vi "Trainging_Program_redesign_Alarm.vi"() -> ()   [LabVIEW 2014]
uses:
  <vilib>/Utility/file.llb/Write To Spreadsheet File (I64).vi
  <vilib>/Utility/file.llb/Write To Spreadsheet File (DBL).vi
  NeuroSky_Dll_Call/Debug/NeuroSky_Dll_Call.dll
panel:
  out "큐사인":bool
  out "실험종료":bool=TRUE
  out "icon_온도":bool
  out "icon_자판":bool
  out "icon_침대":bool
  out "icon_기계":bool
  out "icon_응급":bool=TRUE
  out "icon_용변":bool
  out "error out":errorcluster={"status"=TRUE, "code"=10, "source"="Create Folder in Trainging_Set_For_ LDA_Matrix_RSVP.vi<APPEND>\nC:\\Emotion_Research\\_Training_Test(LDA)\\2014-08-30"}
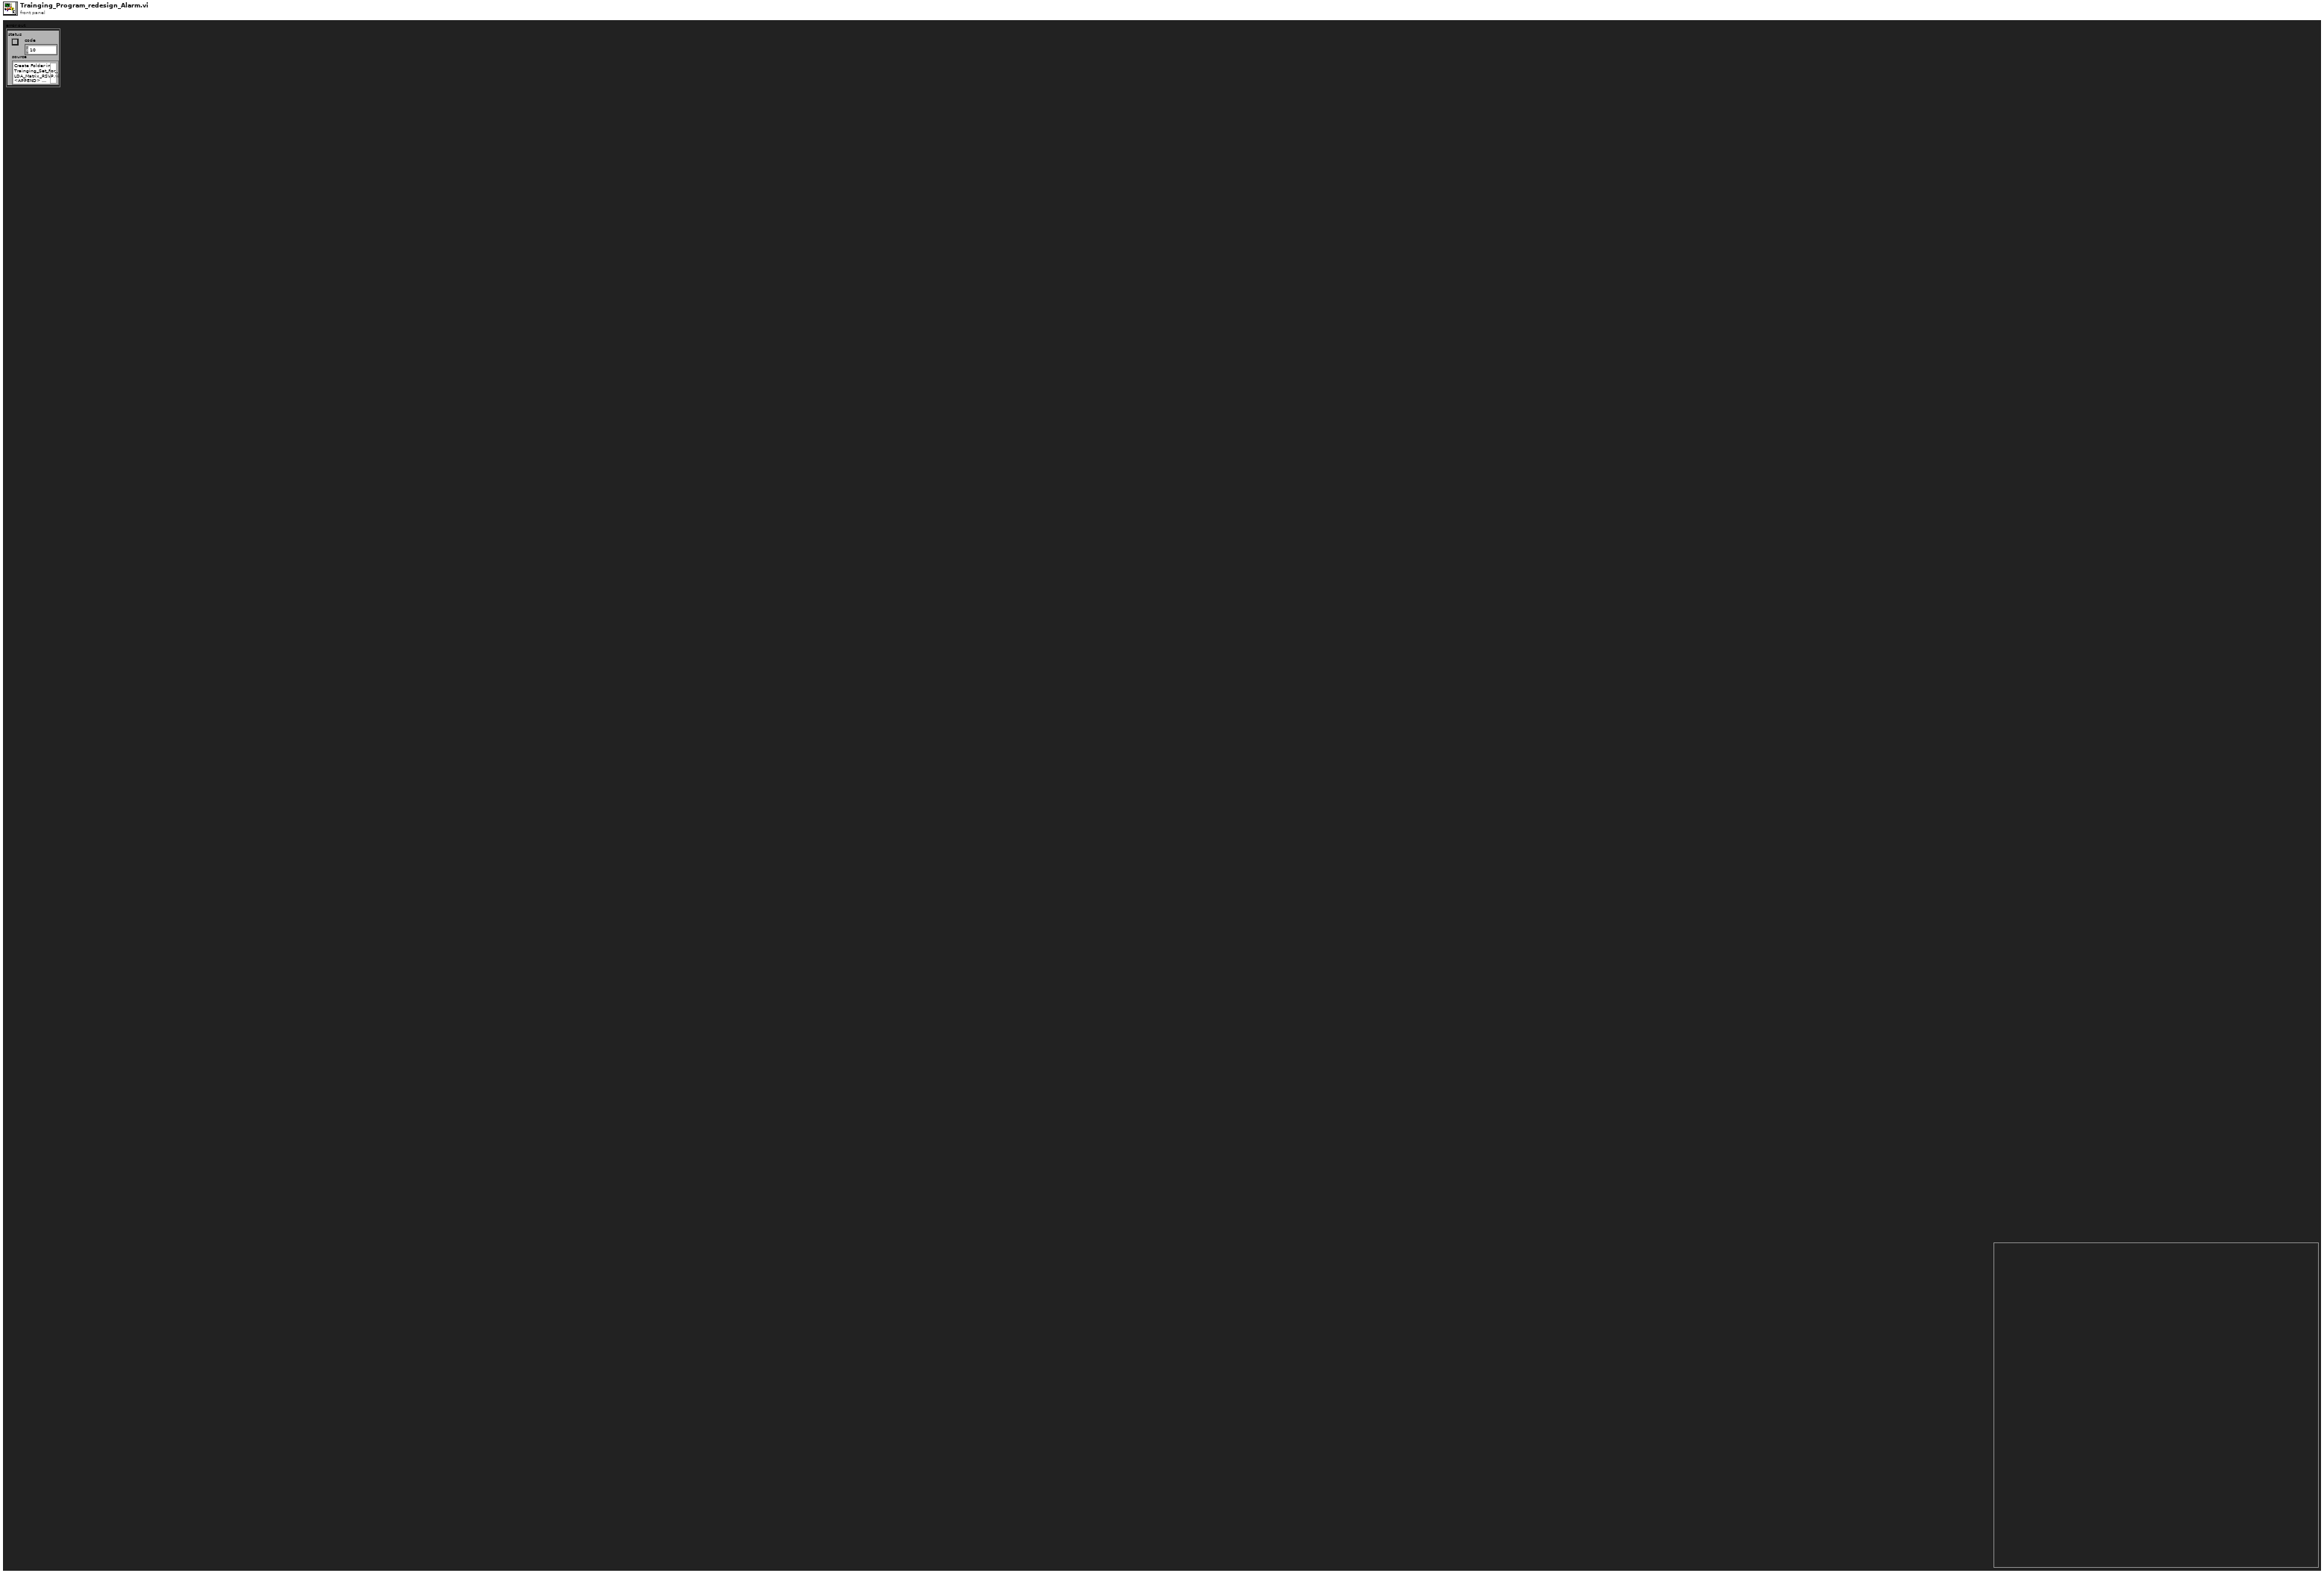
[diagram p1: front panel]
types:
  T1 = typedef "NI_Matrix.lvlib/RealMatrix.ctl" = dbl[][]
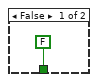
[diagram p2: hidden frame]
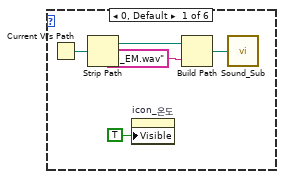
[diagram p3: hidden frame]
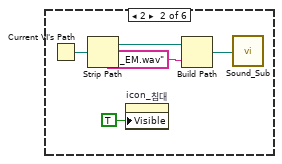
[diagram p4: hidden frame]
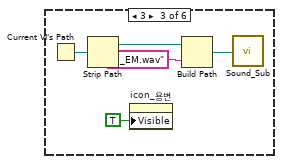
[diagram p5: hidden frame]
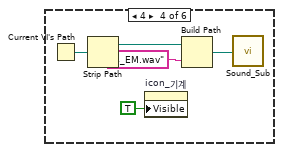
[diagram p6: hidden frame]
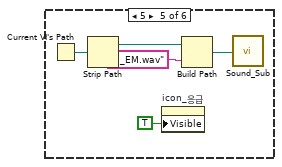
[diagram p7: hidden frame]
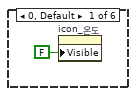
[diagram p8: hidden frame]
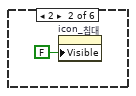
[diagram p9: hidden frame]
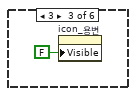
[diagram p10: hidden frame]
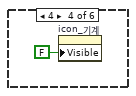
[diagram p11: hidden frame]
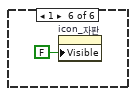
[diagram p12: hidden frame]
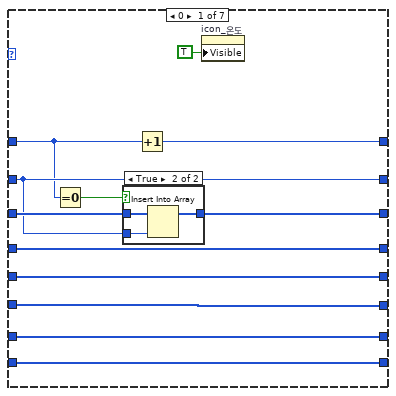
[diagram p14: hidden frame]
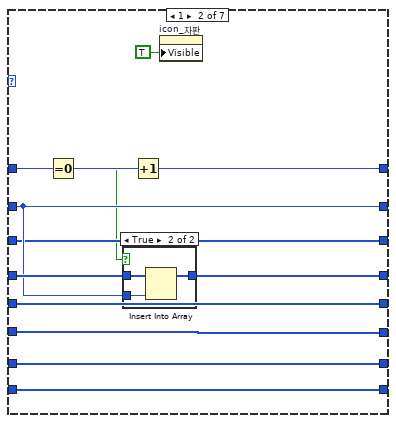
[diagram p16: hidden frame]
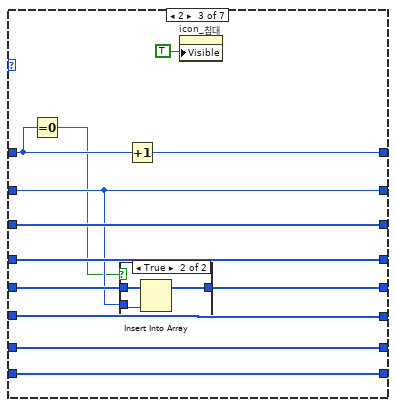
[diagram p18: hidden frame]
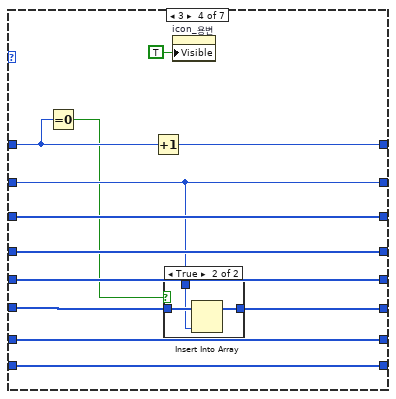
[diagram p20: hidden frame]
diagram:
  w8 = 500 ("Position:Left")
  w1 = FALSE ("Visible")
  # "0 = 온도\n1 = 자판\n2 = 침대\n3 = 용변 \n4 = 기계 \n5 = 응급"
  n1 = property on="icon_기계" class="Bool (strict)"("Left"=w8, "Top"=w8) -> ()  [unwired: 2 in, 2 out]
  n2 = property on="icon_자판" class="Bool (strict)"("Left"=w8, "Top"=w8) -> ()  [unwired: 2 in, 2 out]
  n3 = property on="icon_침대" class="Bool (strict)"("Left"=w8, "Top"=w8) -> ()  [unwired: 2 in, 2 out]
  n4 = property on="icon_응급" class="Bool (strict)"("Left"=w8, "Top"=w8) -> ()  [unwired: 2 in, 2 out]
  n5 = property on="icon_온도" class="Bool (strict)"("Left"=w8, "Top"=w8) -> ()  [unwired: 2 in, 2 out]
  n6 = property on="icon_용변" class="Bool (strict)"("Left"=w8, "Top"=w8) -> ()  [unwired: 2 in, 2 out]
  n7 = property on="실험종료" class="Bool (strict)"("Left"=200 ("Position:Left"), "Top"=600 ("Position:Top")) -> ()  [unwired: 2 in, 2 out]
  n8 = property on="큐사인" class="Bool (strict)"("Left"=w8, "Top"=w8) -> ()  [unwired: 2 in, 2 out]
  n9 = property on="큐사인" class="Bool (strict)"("Visible"=w1) -> ()  [unwired: 2 in, 2 out]
  n10 = property on="실험종료" class="Bool (strict)"("Visible"=w1) -> ()  [unwired: 2 in, 2 out]
  n11 = property on="icon_기계" class="Bool (strict)"("Visible"=w1) -> ()  [unwired: 2 in, 2 out]
  n12 = property on="icon_온도" class="Bool (strict)"("Visible"=w1) -> ()  [unwired: 2 in, 2 out]
  n13 = property on="icon_자판" class="Bool (strict)"("Visible"=w1) -> ()  [unwired: 2 in, 2 out]
  n14 = property on="icon_침대" class="Bool (strict)"("Visible"=w1) -> ()  [unwired: 2 in, 2 out]
  n15 = property on="icon_응급" class="Bool (strict)"("Visible"=w1) -> ()  [unwired: 2 in, 2 out]
  n16 = property on="icon_용변" class="Bool (strict)"("Visible"=w1) -> ()  [unwired: 2 in, 2 out]
  n17 = flat-sequence {
    tunnel: [w32] -> w31
    tunnel: w31 -> [w46]
    tunnel: [w46] -> w30
    tunnel: [w45] -> w29
    tunnel: w30 -> [w62]
    tunnel: w29 -> [w58]
    tunnel: [w62] -> w28
    tunnel: [w52] -> w27
    tunnel: [w57] -> w26
    tunnel: [w56] -> w25
    tunnel: w28 -> [w372]
    tunnel: w27 -> [w369]
    tunnel: w26 -> [w370]
    tunnel: w25 -> [w371]
    tunnel: [w372] -> w24
    tunnel: [w369] -> w23
    tunnel: [w370] -> w22
    tunnel: [w371] -> w21
    tunnel: w24 -> [w390]
    tunnel: w23 -> [w394]
    tunnel: w22 -> [w402]
    tunnel: w21 -> [w401]
    tunnel: [w389] -> w20
    tunnel: [w388] -> w19
    tunnel: [w390] -> w18
    tunnel: [w389] -> w6
    tunnel: [w388] -> w5
    tunnel: w20 -> [w419]
    tunnel: w19 -> [w429]
    tunnel: w18 -> [w414]
    tunnel: [w414] -> w17
    tunnel: w6 -> [w420]
    tunnel: w5 -> [w418]
    tunnel: [w420] -> w4
    tunnel: [w418] -> w3
    tunnel: w17 -> [w441]
    tunnel: w4 -> [w452]
    tunnel: w3 -> [w451]
    frame #0 {
      n18 = Get Date/Time In Seconds() -> (seconds since 1Jan1904=w37:timestamp)
      n19 = global read "Control_Panel_정리.vi" "피험자 이름"() -> (w33:string)
      n20 = Get Date/Time String(seconds (now)=w37) -> (date string=w36:string)  [unwired: 2 in, 1 out]
      n21 = Concatenate Strings("Emotion_Research\\" ("string"), w33, "_Training_Test(LDA)\\" ("문자열")) -> (w41:string)
      n22 = Concatenate Strings(w41, w36) -> (w39:string)
      n23 = Build Path(base path=path "C:/" ("path"), name or relative path=w39) -> (appended path=w38:path)
      n24 = Create Folder(path (use dialog)=w38) -> (created path=w32:path, error out=→"error out":errorcluster)  [unwired: 2 in, 1 out]
    }
    frame #1 {
      n25 = while {
        stop <- w47 stop-if-true
        n26 = global read "Control_Panel_정리.vi" "Start"() -> (w48:bool)
        n27 = case shown="True" w48 {
          tunnel: [FALSE ("Connected") w50] -> w47
          frame False {
          }
          frame True {
            n28 = call "Control_module.vi"("Turn on"=TRUE ("Device Control Enabled")) -> ("Connected"=w50:bool)
            n29 = global write "Control_Panel_정리.vi" "Device Control Enabled"(w50) -> ()
          }
        }
      }
      n30 = global read "Control_Panel_정리.vi" "Experimentation_num"() -> (w44:i32)
      n31 = global read "Control_Panel_정리.vi" "Random_num"() -> (w43:i32)
      n32 = call "Random2.vi"("Random_num"=w43, "전체횟수"=w44) -> ("배열"=w45:i32[])
    }
    frame #2 {
      n33 = global write "Control_Panel_정리.vi" "Acquisition Mode"(TRUE ("Device Control Enabled")) -> ()
      n34 = global write "Control_Panel_정리.vi" "Device Control Enabled"(FALSE ("Device Control Enabled")) -> ()
      n35 = while {
        tunnel: w58 -> [w107]
        shift-right: [w102] -> _
        shift-left: 0 ("y") -> [w103]
        shift-right: [w101] -> w56
        shift-left: i32[] [] ("subarray") -> [w89]
        shift-right: [w99] -> w52
        shift-left: dbl[] [] -> [w100]
        shift-right: [w92] -> w57
        shift-left: i32[][] [] -> [w88]
        i -> [w98]
        stop <- w97 stop-if-true
        # "현재타겟에 해당하는 \nflash order 만 가져옴"
        n36 = flat-sequence {
          tunnel: [w111] -> w78
          tunnel: w107 -> [w113]
          tunnel: w98 -> [w112]
          tunnel: [w114] -> w76
          tunnel: w103 -> [w114]
          tunnel: [w108] -> w74
          tunnel: w78 -> [w147]
          tunnel: [w147] -> w77
          tunnel: w76 -> [w146]
          tunnel: [w146] -> w75
          tunnel: w74 -> [w145]
          tunnel: [w145] -> w73
          tunnel: w77 -> [w157]
          tunnel: [w157] -> w81
          tunnel: w75 -> [w156]
          tunnel: [w156] -> w80
          tunnel: w73 -> [w155]
          tunnel: [w155] -> w79
          tunnel: w81 -> [w161]
          tunnel: [w161] -> w72
          tunnel: w80 -> [w160]
          tunnel: [w160] -> w70
          tunnel: w79 -> [w159]
          tunnel: [w159] -> w68
          tunnel: w72 -> [w179]
          tunnel: [w179] -> w71
          tunnel: w70 -> [w178]
          tunnel: [w178] -> w69
          tunnel: w68 -> [w177]
          tunnel: [w177] -> w67
          tunnel: w71 -> [w197]
          tunnel: w69 -> [w194]
          tunnel: w67 -> [w188]
          tunnel: [w188] -> w85
          tunnel: [w190] -> w84
          tunnel: [w180] -> w83
          tunnel: [w193] -> w82
          tunnel: w85 -> [w361]
          tunnel: w84 -> [w360]
          tunnel: w83 -> [w359]
          tunnel: w82 -> [w358]
          tunnel: [w361] -> w66
          tunnel: [w360] -> w65
          tunnel: [w359] -> w64
          tunnel: [w358] -> w63
          tunnel: [w365] -> w90
          tunnel: [w366] -> w102
          tunnel: [w367] -> w95
          tunnel: [w368] -> w93
          tunnel: w66 -> [w368]
          tunnel: w65 -> [w367]
          tunnel: w64 -> [w366]
          tunnel: w63 -> [w365]
          frame #0 {
            # "타겟 순서"
            # "결과로 만들어지는 배열은 일차원배열로\n출력되면 랜덤 숫자는 0부터 시작함"
            n37 = global read "Control_Panel_정리.vi" "Random_num"() -> (w109:i32)
            n38 = global read "Control_Panel_정리.vi" "Flash_Repeat"() -> (w110:i32)
            n39 = Index Array(array=w113, index=w112) -> (element=w108:i32)
            n40 = case shown="1" w108 {
              frame 0, Default {
                n41 = Current VI's Path() -> (path=w117:path)
                n42 = Strip Path(path=w117) -> (stripped path=w118:path)  [unwired: 1 out]
                n43 = property on="icon_온도" class="Bool (strict)"("Visible"=TRUE) -> ()  [unwired: 2 in, 2 out]
                n44 = Build Path(base path=w118, name or relative path="0_EM.wav" ("이름 또는 상대 경로")) -> (appended path=w116:path)
                n45 = call "Sound_Sub.vi"("path"=w116) -> ()
              }
              frame 2 {
                n46 = Current VI's Path() -> (path=w121:path)
                n47 = Strip Path(path=w121) -> (stripped path=w122:path)  [unwired: 1 out]
                n48 = property on="icon_침대" class="Bool (strict)"("Visible"=TRUE) -> ()  [unwired: 2 in, 2 out]
                n49 = Build Path(base path=w122, name or relative path="2_EM.wav" ("이름 또는 상대 경로")) -> (appended path=w124:path)
                n50 = call "Sound_Sub.vi"("path"=w124) -> ()
              }
              frame 3 {
                n51 = Current VI's Path() -> (path=w126:path)
                n52 = Strip Path(path=w126) -> (stripped path=w127:path)  [unwired: 1 out]
                n53 = property on="icon_용변" class="Bool (strict)"("Visible"=TRUE) -> ()  [unwired: 2 in, 2 out]
                n54 = Build Path(base path=w127, name or relative path="3_EM.wav" ("이름 또는 상대 경로")) -> (appended path=w129:path)
                n55 = call "Sound_Sub.vi"("path"=w129) -> ()
              }
              frame 4 {
                n56 = Current VI's Path() -> (path=w131:path)
                n57 = Strip Path(path=w131) -> (stripped path=w132:path)  [unwired: 1 out]
                n58 = property on="icon_기계" class="Bool (strict)"("Visible"=TRUE) -> ()  [unwired: 2 in, 2 out]
                n59 = Build Path(base path=w132, name or relative path="4_EM.wav" ("이름 또는 상대 경로")) -> (appended path=w134:path)
                n60 = call "Sound_Sub.vi"("path"=w134) -> ()
              }
              frame 5 {
                n61 = Current VI's Path() -> (path=w136:path)
                n62 = Strip Path(path=w136) -> (stripped path=w137:path)  [unwired: 1 out]
                n63 = property on="icon_응급" class="Bool (strict)"("Visible"=TRUE) -> ()  [unwired: 2 in, 2 out]
                n64 = Build Path(base path=w137, name or relative path="5_EM.wav" ("이름 또는 상대 경로")) -> (appended path=w139:path)
                n65 = call "Sound_Sub.vi"("path"=w139) -> ()
              }
              frame 1 {
                n66 = Current VI's Path() -> (path=w142:path)
                n67 = Strip Path(path=w142) -> (stripped path=w143:path)  [unwired: 1 out]
                n68 = property on="icon_자판" class="Bool (strict)"("Visible"=TRUE) -> ()  [unwired: 2 in, 2 out]
                n69 = Build Path(base path=w143, name or relative path="1_EM.wav" ("이름 또는 상대 경로")) -> (appended path=w141:path)
                n70 = call "Sound_Sub.vi"("path"=w141) -> ()
              }
            }
            n71 = call "Random2.vi"("Random_num"=w109, "전체횟수"=w110) -> ("배열"=w111:i32[])
          }
          frame #1 {
            n72 = case shown="5" w145 {
              frame 0, Default {
                n73 = property on="icon_온도" class="Bool (strict)"("Visible"=FALSE) -> ()  [unwired: 2 in, 2 out]
              }
              frame 2 {
                n74 = property on="icon_침대" class="Bool (strict)"("Visible"=FALSE) -> ()  [unwired: 2 in, 2 out]
              }
              frame 3 {
                n75 = property on="icon_용변" class="Bool (strict)"("Visible"=FALSE) -> ()  [unwired: 2 in, 2 out]
              }
              frame 4 {
                n76 = property on="icon_기계" class="Bool (strict)"("Visible"=FALSE) -> ()  [unwired: 2 in, 2 out]
              }
              frame 5 {
                n77 = property on="icon_응급" class="Bool (strict)"("Visible"=FALSE) -> ()  [unwired: 2 in, 2 out]
              }
              frame 1 {
                n78 = property on="icon_자판" class="Bool (strict)"("Visible"=FALSE) -> ()  [unwired: 2 in, 2 out]
              }
            }
          }
          frame #2 {
            n79 = property on="큐사인" class="Bool (strict)"("Visible"=TRUE) -> ()  [unwired: 2 in, 2 out]
          }
          frame #3 {
            # "1. NeuroSky의 경우 전송되지 않은 데이터도 축적하여 FIFO 방식으로 GetValue() 함수를 호출할때 한개의 값씩 보내는 방식을 취한다. 현재 MindWave Mobile은 Sampling rate가 512 Hz이며, 2ms의 wait 를 주어 값을 받을 경우 초당 12 sample씩 데이터가 밀리게 된다 \n\n                512 sample/sec - 500 sample /sec = 12 sample /sec\n\n따라서 wait를 주어 500 sample로 맞추는 방식보다 GetValue를 data 값이 정상으로 나올때까지 while로 지속적으로 호출하는 방식으로 syncrhonize 하는 것이 좋다.\n\n2. NeuroSky가 데이터를 전송하지 않더라고 수집을 하기 때문에 Connect()를 통해 통신이 연결된 후 GetValue()를 통해 값을 호출 할때 GetValue()사이에 시간 간격이 생기면 값이 밀리게 된다. 따라서 값을 호출하지 않는 경우 Disconnect()를 통해 통신을 끊어야 Synchornize를 할 수 있다.\n\n3. 통신을 다시 할 경우 1051개의 쓰레기 데이터를 전송하기 때문에 이 값은 dump해버리도록 한다."
            n80 = global read "Control_Panel_정리.vi" "Connected"() -> (w158:bool)
            n81 = case shown="False" w158 {
              frame False {
                n82 = flat-sequence {
                  frame #0 {
                    n83 = dll-call lib="PTH2uabs CUsersJaehongDesktop연구_programNeuroSky_최종본NeuroSky_Dll_CallDebugNeuroSky_Dll_Call.dll" fn="Connect"() -> ("errCode"=w162:string)  [unwired: 3 in, 2 out]
                    n84 = global write "Control_Panel_정리.vi" "Port Status"(w162) -> ()
                  }
                  frame #1 {
                    n85 = global write "Control_Panel_정리.vi" "Connection"("Reconnected") -> ()
                    n86 = global write "Control_Panel_정리.vi" "Connected"(TRUE ("Connected")) -> ()
                  }
                  frame #2 {
                    n87 = for {
                      N: 1200 -> [_]
                      tunnel: [w167] -> w165 mode=indexing
                      n88 = while {
                        tunnel: [w169] -> w167
                        stop <- w168 stop-if-true
                        n89 = Initialize Array(0.0 ("element"), 100 ("dimension size")) -> (w174:dbl[])
                        n90 = dll-call lib="PTH2uabs CUsersJaehongDesktop연구_programNeuroSky_최종본NeuroSky_Dll_CallDebugNeuroSky_Dll_Call.dll" fn="GetValue"("result"=w174) -> ("result"=w175:dbl[])  [unwired: 4 in, 2 out]
                        n91 = Index Array(array=w175, index=1) -> (element=w169:dbl)
                        n92 = Greater?(x=w169, y=0.0) -> (0:w168:bool)
                      }
                    }
                    n93 = global write "Control_Panel_정리.vi" "Dump"(w165) -> ()
                  }
                }
              }
              frame True {
              }
            }
          }
          frame #4 {
            n94 = property on="큐사인" class="Bool (strict)"("Visible"=FALSE) -> ()  [unwired: 2 in, 2 out]
          }
          frame #5 {
            w189 = i32[] []
            # "random_repeat * random_num"
            # "마지막 자극제시 후\n1초데이터를 받기 위한 부분\n(960ms)"
            n95 = while {
              tunnel: w197 -> [w235]
              shift-right: [w198] -> w193
              shift-left: dbl[] [] -> [w200]
              shift-right: [w234] -> w182
              shift-left: w189 -> [w233]
              shift-right: [w231] -> w183
              shift-left: w189 -> [w232]
              shift-right: [w229] -> w184
              shift-left: w189 -> [w230]
              shift-right: [w227] -> w185
              shift-left: w189 -> [w228]
              shift-right: [w225] -> w186
              shift-left: w189 -> [w226]
              shift-right: [w224] -> w187
              shift-left: w189 -> [w216]
              shift-right: [w222] -> w180
              shift-left: w194 -> [w223]
              shift-right: [w221] -> _
              shift-left: 0 -> [w219]
              shift-right: [w217] -> _
              shift-left: 0 ("y") -> [w218]
              tunnel: 8 -> [w199]
              i -> [w220]
              stop <- w201 stop-if-true
              # "ITR =  ~240ms"
              # "0 = 온도\n1 = 자판\n2 = 침대\n3 = 용변 \n4 = 기계 \n5 = 응급"
              n96 = flat-sequence {
                tunnel: [w346] -> w198
                tunnel: w200 -> [w344]
                frame #0 {
                  # "Packet 단위로 송신\n이는 반짝이는 효과를 주기 위함\n1 Packet = 20 data (~40ms)"
                  n97 = for {
                    N: 20 -> [_]
                    tunnel: [w347] -> w345 mode=indexing
                    n98 = while {
                      tunnel: [w349] -> w347
                      stop <- w348 stop-if-true
                      n99 = Initialize Array(0.0 ("element"), 100 ("dimension size")) -> (w355:dbl[])
                      n100 = dll-call lib="PTH2uabs CUsersJaehongDesktop연구_programNeuroSky_최종본NeuroSky_Dll_CallDebugNeuroSky_Dll_Call.dll" fn="GetValue"("result"=w355) -> ("errCode"=w351:string, "result"=w356:dbl[])  [unwired: 3 in, 2 out]
                      n101 = global write "Control_Panel_정리.vi" "Value Achieving Status"(w351) -> ()
                      n102 = Index Array(array=w356, index=1) -> (element=w349:dbl)
                      n103 = Greater?(x=w349, y=-100000.0) -> (0:w348:bool)
                    }
                    n104 = global write "Control_Panel_정리.vi" "웨이브폼 차트"(w347) -> ()
                  }
                  n105 = Build Array (concatenate)(w344, w345) -> (w346:dbl[])
                }
              }
              n106 = global read "Control_Panel_정리.vi" "Random_num"() -> (w203:i32)
              n107 = global read "Control_Panel_정리.vi" "Flash_Repeat"() -> (w204:i32)
              n108 = Increment(x=w220) -> (x+1=w206:i32)
              n109 = Quotient & Remainder(x=w206, y=6) -> (x-y*floor(x/y)=w211:i32)  [unwired: 1 out]
              n110 = Equal To 0?(x=w211) -> (x = 0?=w209:bool)
              n111 = Multiply(x=w204, y=w203) -> (x*y=w202:i32)
              n112 = Add(x=w199, y=w202) -> (x+y=w215:i32)
              n113 = Greater Or Equal?(x=w219, y=w202) -> (x >= y?=w208:bool)
              n114 = Increment(x=w219) -> (x+1=w210:i32)
              n115 = Increment(x=w223) -> (x+1=w213:i32)
              n116 = Equal?(x=w219, y=w215) -> (x = y?=w201:bool)
              n117 = Index Array(array=w235, index=w219) -> (element=w205:i32)
              n118 = Or(x=w209, y=w208) -> (x .or. y?=w207:bool)
              n119 = Select(t=w210, s=w209, f=w219) -> (s? t:f=w221:i32)
              n120 = Select(t=w203, s=w207, f=w205) -> (s? t:f=w214:i32)
              n121 = case shown="6, Default" w214 {
                tunnel: w213 -> [w241 w257 w272 w288 w304 w321 w336]
                tunnel: [w246 w254 w279 w295 w311 w327 w342] -> w234
                tunnel: w233 -> [w247 w254 w279 w295 w311 w327 w342]
                tunnel: w232 -> [w245 w263 w276 w292 w308 w325 w341]
                tunnel: [w245 w262 w276 w292 w308 w325 w341] -> w231
                tunnel: w230 -> [w244 w261 w278 w291 w307 w324 w340]
                tunnel: [w244 w261 w277 w291 w307 w324 w340] -> w229
                tunnel: w228 -> [w243 w260 w275 w294 w306 w323 w339]
                tunnel: [w243 w260 w275 w293 w306 w323 w339] -> w227
                tunnel: w226 -> [w242 w259 w274 w290 w310 w322 w338]
                tunnel: [w242 w259 w274 w290 w309 w322 w338] -> w225
                tunnel: w216 -> [w238 w258 w273 w289 w305 w326 w337]
                tunnel: [w238 w258 w273 w289 w305 w318 w337] -> w224
                tunnel: [w241 w257 w272 w288 w304 w321 w336] -> w222
                tunnel: w218 -> [w240 w256 w271 w286 w303 w319 _]
                tunnel: [w239 w255 w270 w287 w302 w320 0] -> w217
                frame 0 {
                  n122 = Equal To 0?(x=w240) -> (x = 0?=w236:bool)
                  n123 = case shown="True" w236 {
                    tunnel: w247 -> [w248 w251]
                    tunnel: [w248 w250] -> w246
                    tunnel: w241 -> [_ w249]
                    frame False {
                    }
                    frame True {
                      n124 = Insert Into Array(array=w251, new element=w249) -> (w250:i32[])  [unwired: 1 in]
                    }
                  }
                  n125 = Increment(x=w240) -> (x+1=w239:i32)
                  n126 = property on="icon_온도" class="Bool (strict)"("Visible"=TRUE) -> ()  [unwired: 2 in, 2 out]
                }
                frame 1 {
                  n127 = Equal To 0?(x=w256) -> (x = 0?=w252:bool)
                  n128 = case shown="True" w252 {
                    tunnel: w263 -> [w264 w267]
                    tunnel: [w264 w266] -> w262
                    tunnel: w257 -> [_ w265]
                    frame False {
                    }
                    frame True {
                      n129 = Insert Into Array(array=w267, new element=w265) -> (w266:i32[])  [unwired: 1 in]
                    }
                  }
                  n130 = Increment(x=w256) -> (x+1=w255:i32)
                  n131 = property on="icon_자판" class="Bool (strict)"("Visible"=TRUE) -> ()  [unwired: 2 in, 2 out]
                }
                frame 2 {
                  n132 = Equal To 0?(x=w271) -> (x = 0?=w268:bool)
                  n133 = case shown="True" w268 {
                    tunnel: w278 -> [w280 w283]
                    tunnel: [w280 w282] -> w277
                    tunnel: w272 -> [_ w281]
                    frame False {
                    }
                    frame True {
                      n134 = Insert Into Array(array=w283, new element=w281) -> (w282:i32[])  [unwired: 1 in]
                    }
                  }
                  n135 = Increment(x=w271) -> (x+1=w270:i32)
                  n136 = property on="icon_침대" class="Bool (strict)"("Visible"=TRUE) -> ()  [unwired: 2 in, 2 out]
                }
                frame 3 {
                  n137 = Equal To 0?(x=w286) -> (x = 0?=w284:bool)
                  n138 = Increment(x=w286) -> (x+1=w287:i32)
                  n139 = case shown="True" w284 {
                    tunnel: w294 -> [w296 w299]
                    tunnel: [w296 w298] -> w293
                    tunnel: w288 -> [_ w297]
                    frame False {
                    }
                    frame True {
                      n140 = Insert Into Array(array=w299, new element=w297) -> (w298:i32[])  [unwired: 1 in]
                    }
                  }
                  n141 = property on="icon_용변" class="Bool (strict)"("Visible"=TRUE) -> ()  [unwired: 2 in, 2 out]
                }
                frame 4 {
                  n142 = Equal To 0?(x=w303) -> (x = 0?=w300:bool)
                  n143 = case shown="False" w300 {
                    tunnel: w310 -> [w312 w315]
                    tunnel: [w312 w314] -> w309
                    tunnel: w304 -> [_ w313]
                    frame False {
                    }
                    frame True {
                      n144 = Insert Into Array(array=w315, new element=w313) -> (w314:i32[])  [unwired: 1 in]
                    }
                  }
                  n145 = Increment(x=w303) -> (x+1=w302:i32)
                  n146 = property on="icon_기계" class="Bool (strict)"("Visible"=TRUE) -> ()  [unwired: 2 in, 2 out]
                }
                frame 5 {
                  n147 = Equal To 0?(x=w319) -> (x = 0?=w316:bool)
                  n148 = Increment(x=w319) -> (x+1=w320:i32)
                  n149 = property on="icon_응급" class="Bool (strict)"("Visible"=TRUE) -> ()  [unwired: 2 in, 2 out]
                  n150 = case shown="True" w316 {
                    tunnel: w326 -> [w328 w331]
                    tunnel: [w328 w330] -> w318
                    tunnel: w321 -> [_ w329]
                    frame False {
                    }
                    frame True {
                      n151 = Insert Into Array(array=w331, new element=w329) -> (w330:i32[])  [unwired: 1 in]
                    }
                  }
                }
                frame 6, Default {
                  w333 = FALSE ("Visible")
                  w332 = FALSE ("Visible")
                  w334 = FALSE ("Visible")
                  n152 = property on="icon_응급" class="Bool (strict)"("Visible"=w334) -> ()  [unwired: 2 in, 2 out]
                  n153 = property on="icon_용변" class="Bool (strict)"("Visible"=w334) -> ()  [unwired: 2 in, 2 out]
                  n154 = property on="icon_기계" class="Bool (strict)"("Visible"=w332) -> ()  [unwired: 2 in, 2 out]
                  n155 = property on="icon_온도" class="Bool (strict)"("Visible"=w332) -> ()  [unwired: 2 in, 2 out]
                  n156 = property on="icon_침대" class="Bool (strict)"("Visible"=w333) -> ()  [unwired: 2 in, 2 out]
                  n157 = property on="icon_자판" class="Bool (strict)"("Visible"=w333) -> ()  [unwired: 2 in, 2 out]
                }
              }
            }
            n158 = Build Array(w182, w183, w184, w185, w186, w187) -> (w195:i32[][])
            n159 = Transpose 2D Array(2D array=w195) -> (transposed array=w190:i32[][])
          }
          frame #6 {
            # "1 Iteration이 끝나고 Disconnect하도록 한다. Synchronize를 위한 방법론"
            n160 = global read "Control_Panel_정리.vi" "Connected"() -> (w357:bool)
            n161 = case shown="True" w357 {
              frame False {
              }
              frame True {
                n162 = flat-sequence {
                  frame #0 {
                    n163 = dll-call lib="PTH2uabs CUsersJaehongDesktop연구_programNeuroSky_최종본NeuroSky_Dll_CallDebugNeuroSky_Dll_Call.dll" fn="Disconnect"() -> ()  [unwired: 4 in, 2 out]
                  }
                  frame #1 {
                    n164 = global write "Control_Panel_정리.vi" "Connection"("Disconnected") -> ()
                    n165 = global write "Control_Panel_정리.vi" "Connected"(FALSE ("Connected")) -> ()
                  }
                }
              }
            }
          }
          frame #7 {
            w364 = FALSE ("Visible")
            n166 = property on="icon_자판" class="Bool (strict)"("Visible"=w364) -> ()  [unwired: 2 in, 2 out]
            n167 = property on="icon_기계" class="Bool (strict)"("Visible"=w364) -> ()  [unwired: 2 in, 2 out]
            n168 = property on="icon_침대" class="Bool (strict)"("Visible"=w364) -> ()  [unwired: 2 in, 2 out]
            n169 = property on="icon_응급" class="Bool (strict)"("Visible"=w364) -> ()  [unwired: 2 in, 2 out]
            n170 = property on="icon_온도" class="Bool (strict)"("Visible"=w364) -> ()  [unwired: 2 in, 2 out]
            n171 = property on="icon_용변" class="Bool (strict)"("Visible"=w364) -> ()  [unwired: 2 in, 2 out]
          }
        }
        n172 = global read "Control_Panel_정리.vi" "Experimentation_num"() -> (w87:i32)
        n173 = global read "Control_Panel_정리.vi" "Random_num"() -> (w86:i32)
        n174 = Multiply(x=w87, y=w86) -> (x*y=w105:i32)
        n175 = Subtract(x=w105, y=2) -> (x-y=w106:i32)
        n176 = Greater?(x=w98, y=w106) -> (0:w97:bool)
        n177 = Index Array(array=w95, index (col)=w93) -> (element=w96:i32[])  [unwired: 1 in]
        n178 = Insert Into Array(array=w100, new element=w90) -> (w99:dbl[])  [unwired: 1 in]
        n179 = Delete From Array(array=w95, length=1 ("길이"), index (col)=w93) -> (array with subset deleted=w94:i32[][])  [unwired: 1 in, 1 out]
        n180 = Build Array (concatenate)(w88, w94) -> (w92:i32[][])
        n181 = Insert Into Array(array=w89, new element=w96) -> (w101:i32[])  [unwired: 1 in]
      }
    }
    frame #3 {
      # "현재타겟에 해당하는 \nflash order 만 가져옴"
      # "target=stimulus 때의 order만 가져옴"
      n182 = flat-sequence {
        frame #0 {
          n183 = dll-call lib="PTH2uabs CUsersJaehongDesktop연구_programNeuroSky_최종본NeuroSky_Dll_CallDebugNeuroSky_Dll_Call.dll" fn="FreeConnection"() -> ()  [unwired: 4 in, 2 out]
        }
        frame #1 {
          n184 = property on="실험종료" class="Bool (strict)"("Visible"=TRUE) -> ()  [unwired: 2 in, 2 out]
        }
        frame #2 {
          n185 = global write "Control_Panel_정리.vi" "Value Achieving Status"("All Connection terminated,\nExperiment over" ("name or relative path")) -> ()
          n186 = global write "Control_Panel_정리.vi" "Acquisition Mode"(FALSE ("Device Control Enabled")) -> ()
        }
      }
      n187 = Build Path(base path=w372, name or relative path="Brain.txt") -> (appended path=w375:path)
      n188 = Build Path(base path=w372, name or relative path="Target_order.txt") -> (appended path=w378:path)
      n189 = call-poly <vilib>:"Write To Spreadsheet File.vi"("transpose? (no:F)"=TRUE, "1D data"=w371, "file path (dialog if empty)"=w378) -> ()  [unwired: 5 in, 1 out]
      n190 = Build Path(base path=w372, name or relative path="Nontarget_order.txt") -> (appended path=w379:path)
      n191 = call-poly <vilib>:"Write To Spreadsheet File.vi"("format (%.3f)"="%.6f", "1D data"=w369, "file path (dialog if empty)"=w375) -> ()  [unwired: 5 in, 1 out]
      n192 = call-poly <vilib>:"Write To Spreadsheet File.vi"("transpose? (no:F)"=FALSE, "2D data"=w370, "file path (dialog if empty)"=w379) -> ()  [unwired: 5 in, 1 out]
    }
    frame #4 {
      n193 = global read "Control_Panel_정리.vi" "Experimentation_num"() -> (w405:i32)
      n194 = global read "Control_Panel_정리.vi" "Flash_Repeat"() -> (w407:i32)
      n195 = global read "Control_Panel_정리.vi" "Random_num"() -> (w406:i32)
      n196 = global write "Control_Panel_정리.vi" "Communication Stopped"(TRUE ("Device Control Enabled")) -> ()
      n197 = global read "Control_Panel_정리.vi" "Frame Length"() -> (w403:i32)
      n198 = global read "Control_Panel_정리.vi" "rate"() -> (w404:dbl)
      n199 = call "Subvi_Training_Baseline_w_range_w_weight.vi"("Nontarget_Flash_Order"=w402, "Target_Flash_Order"=w401, "samples per channel"=w403, "Brain_data_source"=w394, "rate"=w404, "Experimentation_num"=w405, "Random_num"=w406, "Random_Repeat"=w407) -> ("Target_ERP"=w385:dbl[], "NonTarget"=w388:dbl[][], "Nontarget_ERP"=w386:dbl[], "Target"=w389:dbl[][])
      n200 = Build Path(base path=w390, name or relative path="Nontarget_ERP_AVG.txt") -> (appended path=w392:path)
      n201 = Build Path(base path=w390, name or relative path="Target_ERP_AVG.txt") -> (appended path=w409:path)
      n202 = Build Path(base path=w390, name or relative path="ERP_Parameters_of_Target_prior.txt") -> (appended path=w399:path)
      n203 = Build Path(base path=w390, name or relative path="ERP_Parameters_of_NonTarget_prior.txt") -> (appended path=w396:path)
      n204 = call-poly <vilib>:"Write To Spreadsheet File.vi"("format (%.3f)"="%.6f", "1D data"=w386, "file path (dialog if empty)"=w392) -> ()  [unwired: 5 in, 1 out]
      n205 = call-poly <vilib>:"Write To Spreadsheet File.vi"("format (%.3f)"="%.6f", "1D data"=w385, "file path (dialog if empty)"=w409) -> ()  [unwired: 5 in, 1 out]
      n206 = call-poly <vilib>:"Write To Spreadsheet File.vi"("format (%.3f)"="%.6f", "2D data"=w389, "file path (dialog if empty)"=w399) -> ()  [unwired: 5 in, 1 out]
      n207 = call-poly <vilib>:"Write To Spreadsheet File.vi"("format (%.3f)"="%.6f", "2D data"=w388, "file path (dialog if empty)"=w396) -> ()  [unwired: 5 in, 1 out]
    }
    frame #5 {
      n208 = Array Size(array=w419) -> (size(s)=w432:i32[])
      n209 = Array Size(array=w429) -> (size(s)=w433:i32[])
      n210 = Index Array(array=w432) -> (element=w434:i32)  [unwired: 1 in]
      n211 = Index Array(array=w433) -> (element=w435:i32)  [unwired: 1 in]
      n212 = for {
        N: w435 -> [_]
        tunnel: [1] -> w437 mode=indexing
      }
      n213 = for {
        N: w434 -> [_]
        tunnel: [0] -> w436 mode=indexing
      }
      n214 = Build Array (concatenate)(w436, w437) -> (w428:i32[])
      n215 = Build Array (concatenate)(w419, w429) -> (w430:dbl[][])
      n216 = global read "Control_Panel_정리.vi" "EEG_Channel_Num"() -> (w411:i32)
      n217 = Insert Into Array(array=w430, index (col)=0 ("비활성화된 인덱스 (열)"), new element=w428) -> (w424:dbl[][])  [unwired: 1 in]
      n218 = call "Subvi_Training_LDA.vi"("Input_Data"=w424) -> ("A * B 2"=w422:T1, "A * B"=w423:T1)
      n219 = Initialize Array(0.090909 ("element"), w411) -> (w413:dbl[])
      n220 = Build Array (concatenate)(w423, w422) -> (w421:T1)
      n221 = Build Path(base path=w414, name or relative path="Weight_Vector_prior.txt") -> (appended path=w417:path)
      n222 = Build Path(base path=w414, name or relative path="LDA_Matrix_Value_prior.txt") -> (appended path=w426:path)
      n223 = call-poly <vilib>:"Write To Spreadsheet File.vi"("format (%.3f)"="%.6f", "1D data"=w413, "file path (dialog if empty)"=w417) -> ()  [unwired: 5 in, 1 out]
      n224 = call-poly <vilib>:"Write To Spreadsheet File.vi"("format (%.3f)"="%.6f", "2D data"=w421, "file path (dialog if empty)"=w426) -> ()  [unwired: 5 in, 1 out]
    }
    frame #6 {
      (unwired) "%.6f" ("format (%.3f)")
      # "addpath('C:\\Users\\Jaehong\\Desktop\\연구_program\\libsvm-3.18\\matlab');"
      n225 = call "SWLDA_통합버전용.vi"("premove"=0.05, "penter"=0.01, "ERP_Nontarget"=w451, "ERP_Target"=w452) -> ("in"=w440:dbl[], "LDA_matrix"=w456:T1)  [unwired: 5 in, 1 out]
      n226 = global read "Control_Panel_정리.vi" "EEG_Channel_Num"() -> (w445:i32)
      n227 = global read "Control_Panel_정리.vi" "EEG_Channel_Num"() -> (w455:i32)
      n228 = global read "Control_Panel_정리.vi" "Random_num"() -> (w454:i32)
      n229 = global read "Control_Panel_정리.vi" "Experimentation_num"() -> (w453:i32)
      n230 = Initialize Array(0.090909 ("element"), w445) -> (w447:dbl[])
      n231 = script code="%addpath to the libsvm toolbox\n\naddpath('C:\\Users\\Server\\Desktop\\NeuroSky\\RSVP_NeuroSky\\libsvm-3.18\\matlab');\n\n%read data set(training)\n\nrow_num = chan_num*4;\ncol_num = icon_num*exp_num;\n\nWeight = Weight';\nnonzeros = find(Weight, row_num);\ntarget = reshape(target', row_num, col_num);\ntarget = target.*Weight(:,ones(1,col_num));\ntarget = target(nonzeros,:);\nnontarget = reshape(nontarget', row_num, col_num);\nnontarget = nontarget.*Weight(:,ones(1,col_num));\nnontarget = nontarget(nonzeros,:);\nEEG_train = [target';nontarget']';\nlength = size(target,2);\ntrainLabel = [ones(length,1);-ones(length, 1)];\n\n% Train the SVM\n\nmodel = ...\nsvmtrain(trainLabel, [(1:col_num*2)' EEG_train'*EEG_train], '-c 1 -g 0.07 -b 1 -t 4 -q');\n\n%save model file\nsvm_savemodel(model,'C:\\WORK\\svm_model.model');" ("Script Node")("Weight"=w440, "target"=w451, "nontarget"=w452, "icon_num"=w454, "chan_num"=w455, "exp_num"=w453) -> ()  [unwired: 1 in, 1 out]
      n232 = Build Path(base path=w441, name or relative path="LDA_Matrix_Value_SWLDA.txt") -> (appended path=w459:path)
      n233 = Build Path(base path=w441, name or relative path="in_SWLDA.txt") -> (appended path=w444:path)
      n234 = Build Path(base path=w441, name or relative path="Weight_Vector_SWLDA.txt") -> (appended path=w450:path)
      n235 = call-poly <vilib>:"Write To Spreadsheet File.vi"("2D data"=w456, "file path (dialog if empty)"=w459) -> ()  [unwired: 6 in, 1 out]
      n236 = call-poly <vilib>:"Write To Spreadsheet File.vi"("format (%.3f)"="%.6f", "1D data"=w440, "file path (dialog if empty)"=w444) -> ()  [unwired: 5 in, 1 out]
      n237 = call-poly <vilib>:"Write To Spreadsheet File.vi"("format (%.3f)"="%.6f", "1D data"=w447, "file path (dialog if empty)"=w450) -> ()  [unwired: 5 in, 1 out]
    }
    frame #7 {
      n238 = global write "Control_Panel_정리.vi" "Communication Stopped"(FALSE ("Device Control Enabled")) -> ()
    }
  }
  "icon_온도" <- FALSE ("icon_전원 6")
  "icon_용변" <- FALSE ("icon_전체종료")
  "icon_자판" <- FALSE ("icon_음량업 2")
  "icon_응급" <- FALSE ("icon_채널다운")
  "icon_기계" <- FALSE ("icon_음량다")
  "icon_침대" <- FALSE ("icon_채널업")
  "실험종료" <- TRUE ("Boolean")
  "큐사인" <- FALSE ("icon_전원 7")
